vi "asset.update_free.vi"(8 "error in":errorcluster, 11 "AssetUpdateStaging in":refnum<class "AssetUpdateStaging.lvclass">) -> (0 "error out":errorcluster, 3 "AssetUpdateStaging out":refnum<class "AssetUpdateStaging.lvclass">)   [LabVIEW 2020, in "AssetUpdateStaging.lvclass"]
doc: "Releases the handle and its associated resources."
uses:
  AssetUpdateStaging.lvclass
  AssetUpdateStaging.lvclass/AssetUpdateStaging.ctl
  client.lvlib
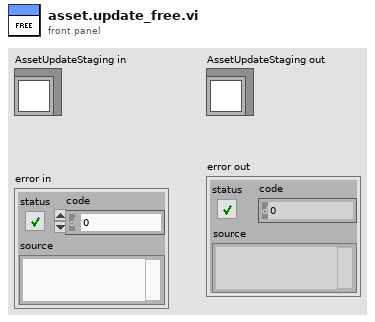
[diagram p1: front panel]
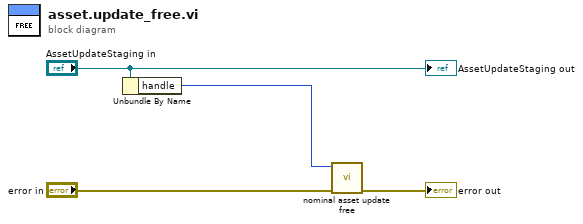
[diagram p0: block diagram]
diagram:
  n1 = Unbundle By Name("AssetUpdateStaging in") -> ("handle"=w2:i32)
  n2 = call "nominal asset update free.vi"("error in (no error)"="error in", "staging"=w2) -> ("error out"=→"error out":errorcluster)  [unwired: 8 in, 1 out]
  "AssetUpdateStaging out" <- "AssetUpdateStaging in"
